vi "Dashboard-Cory.vi"(0 "SensorInputData":T8, 1 "ActuatorInputs":T7, 2 "HMI to Control":T5={"RightDriveValue"=0.0, "LeftDriveValue"=0.0, "Arm Manual "=0.0, "Stacker Manual "=0.0, "Claw Manual "=0.0, "ClawSlightOpenNumber"=0, "Intake Value "=0.0, "Arm States"=enum."4 Tote", "Claw States"=enum."Claw Manual ", "Intake Man. or Sense"=enum."Sensing", "Stacker in Manual?"=FALSE, "Drop Stack? "=FALSE, "Tusk Up Request"=FALSE, "Tusk Down Request"=FALSE, "Inver. Wheels  In Request"=FALSE, "Inverse. Wheels Out Request "=FALSE, "Get Out of Manual Control"=FALSE, "Exit Score State"=FALSE, "DriveStraight Help?"=FALSE, "Stacker Shut Off No."=0, "Stacker Need Off?"=FALSE, "Collecting?"=FALSE, "Go to Hover"=FALSE, "Stack Clamp Lock "=FALSE, "Stack Clamp Unlock "=FALSE, "Claw Intake Value "=0.0, "Stack Clamp Lock No. "=0, "Steal Can (ruin their day?)"=FALSE, "Retract (have mercy?)"=FALSE, "Can Grab No. "=0, "Wench Value to Control "=0.0}, 3 "Stacker to Dashboard":T1={"# of Totes Out"=0, "Stacker State to Index"=enum."Hold", "Stacker Off?"=FALSE, "Stack Clamp Locked?"=FALSE}) -> ()   [LabVIEW 2014]
uses:
  Typedefs/SensorInputData.ctl
  Typedefs/ActuatorInputs.ctl
  Typedefs/HMI_to_Control.ctl
  Typedefs/Arm States.ctl
  Typedefs/ClawStates.ctl
  Typedefs/IntakeWheelSenseOrManual.ctl
  Typedefs/StackerStates.ctl
  Typedefs/StackerToDashboardData.ctl
  <vilib>/Rock Robotics/Network Tables/SD Write Boolean.vi
  <vilib>/Rock Robotics/Network Tables/SD Write Number.vi
  Gensubs/Bert_or_Ernie.vi
  Auton/scriptlib/auto_data.vi
  <vilib>/Rock Robotics/Network Tables/SD Write String Array.vi
panel:
  out "Stack Clamp Locked?":bool
  out "On Bert?":bool
  out "Intake":dbl
  out "Arm":dbl
  out "Stacker":dbl
  out "LeftDrive":dbl
  out "RightDrive":dbl
  out "Stacker Off?":bool
  out "Stacker State to Index":T2=enum."Hold"
  out "Intake See Tote":bool
  out "Claw Manual?":bool=TRUE
  out "Compressor Enabled":bool
  out "Compressor Run":bool
  out "Claw Sees Can":bool
  out "Arm States":T3
  out "Claw States":T4
  in  "MaxSlightOpenNumber":i8
  out "Stacker Manual":bool
  out "# of Totes":u8
  out "Intake Sensing?":bool
  out "ClawOpen%":dbl(slide) scale=0.0..1.0
  out "Tusk":bool
  out "Stacker See Tote":bool
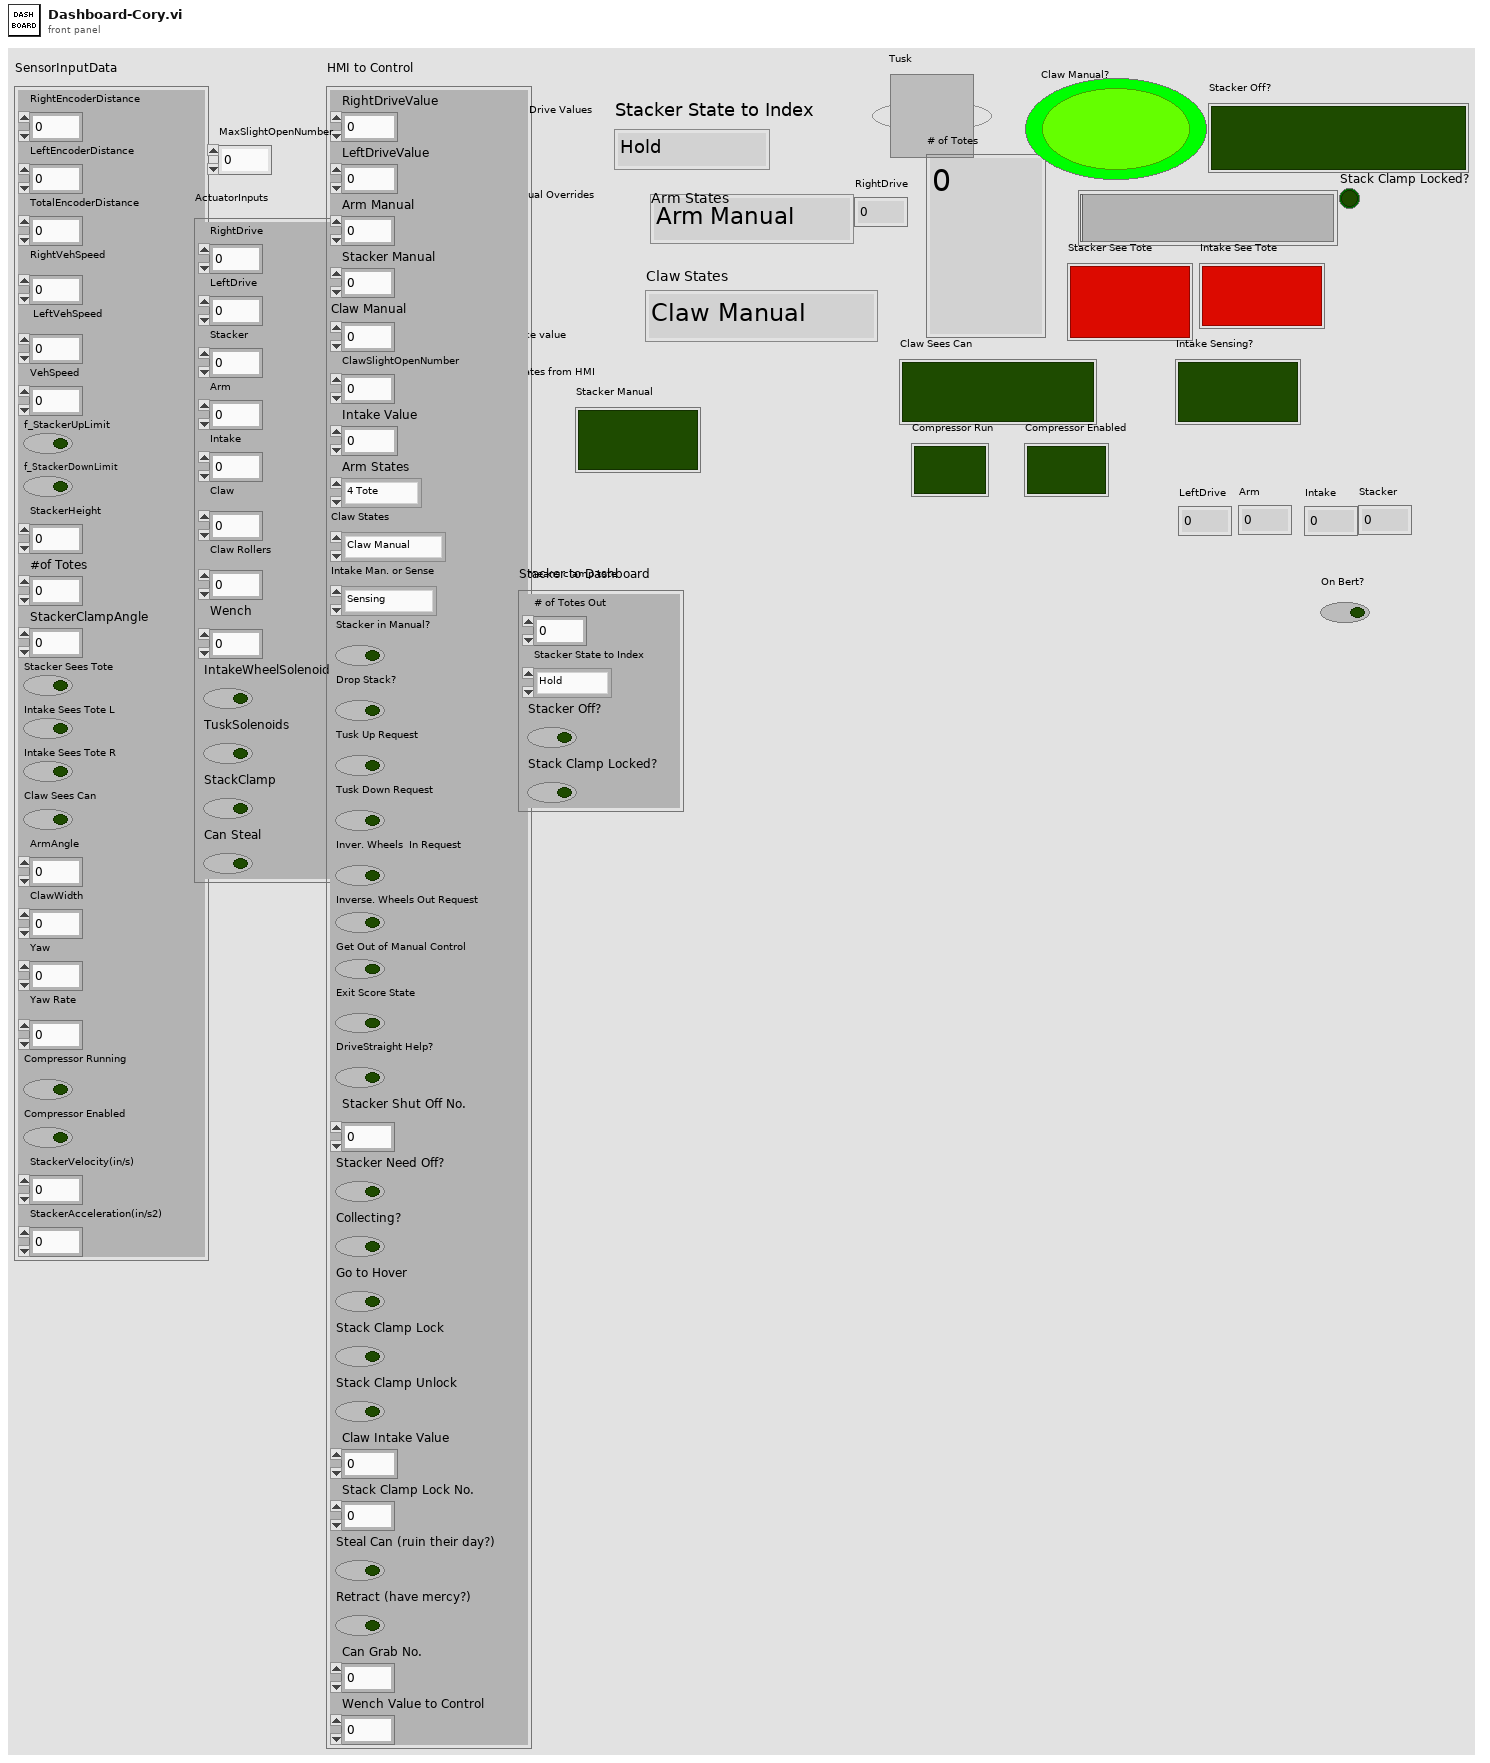
[diagram p1: front panel]
types:
  T1 = typedef "StackerToDashboardData.ctl" = cluster{"# of Totes Out":i32, "Stacker State to Index":T2, "Stacker Off?":bool, "Stack Clamp Locked?":bool}
  T2 = typedef "StackerStates.ctl" = enum16{"Manual ", "Hold", "Hold5", "Hold6", "GetTote", "DropStack", "Hover", "Hover5", "Wait for Up", "DecideHold", "DownTimerPeriod", "Prep Intake for Drop", "Check Arm before 5", "Make Arm ready for 5", "Check Arm before 6", "Make Arm ready for 6", "Delay for 5", "Delay for 6"}
  T3 = typedef "Arm States.ctl" = enum16{"Arm Manual ", "Ground", "Step", "1 Tote", "2 Tote", "3 Tote", "4 Tote", "5 Tote", "6 Tote", "Flip Can Arm", "Grab Can in auto", "Nudge"}
  T4 = typedef "ClawStates.ctl" = enum16{"Claw Manual ", "Claw Open", "Claw Closed", "Claw Slight Open", "Flip Can"}
  T5 = typedef "HMI_to_Control.ctl" = cluster{"RightDriveValue":dbl, "LeftDriveValue":dbl, "Arm Manual ":dbl, "Stacker Manual ":dbl, "Claw Manual ":dbl, "ClawSlightOpenNumber":i8, "Intake Value ":sgl, "Arm States":T3, "Claw States":T4, "Intake Man. or Sense":T6, "Stacker in Manual?":bool, "Drop Stack? ":bool, "Tusk Up Request":bool, "Tusk Down Request":bool, "Inver. Wheels  In Request":bool, "Inverse. Wheels Out Request ":bool, "Get Out of Manual Control":bool, "Exit Score State":bool, "DriveStraight Help?":bool, "Stacker Shut Off No.":i8, "Stacker Need Off?":bool, "Collecting?":bool, "Go to Hover":bool, "Stack Clamp Lock ":bool, "Stack Clamp Unlock ":bool, "Claw Intake Value ":sgl, "Stack Clamp Lock No. ":i8, "Steal Can (ruin their day?)":bool, "Retract (have mercy?)":bool, "Can Grab No. ":i8, "Wench Value to Control ":dbl}
  T6 = typedef "IntakeWheelSenseOrManual.ctl" = enum16{"Sensing", "Manual "}
  T7 = typedef "ActuatorInputs.ctl" = cluster{"RightDrive":dbl, "LeftDrive":dbl, "Stacker":dbl, "Arm":dbl, "Intake":sgl, "Claw":dbl, "Claw Rollers":i8, "Wench":dbl, "IntakeWheelSolenoids":bool, "TuskSolenoids":bool, "StackClamp":bool, "Can Steal":bool}
  T8 = typedef "SensorInputData.ctl" = cluster{"RightEncoderDistance":dbl, "LeftEncoderDistance":dbl, "TotalEncoderDistance":dbl, "RightVehSpeed":dbl, "LeftVehSpeed":dbl, "VehSpeed":dbl, "f_StackerUpLimit":bool, "f_StackerDownLimit":bool, "StackerHeight":dbl, "#of Totes":u8, "StackerClampAngle":dbl, "Stacker Sees Tote":bool, "Intake Sees Tote L":bool, "Intake Sees Tote R":bool, "Claw Sees Can":bool, "ArmAngle":dbl, "ClawWidth":dbl, "Yaw":dbl, "Yaw Rate":dbl, "Compressor Running":bool, "Compressor Enabled":bool, "StackerVelocity(in/s)":dbl, "StackerAcceleration(in/s2)":dbl}
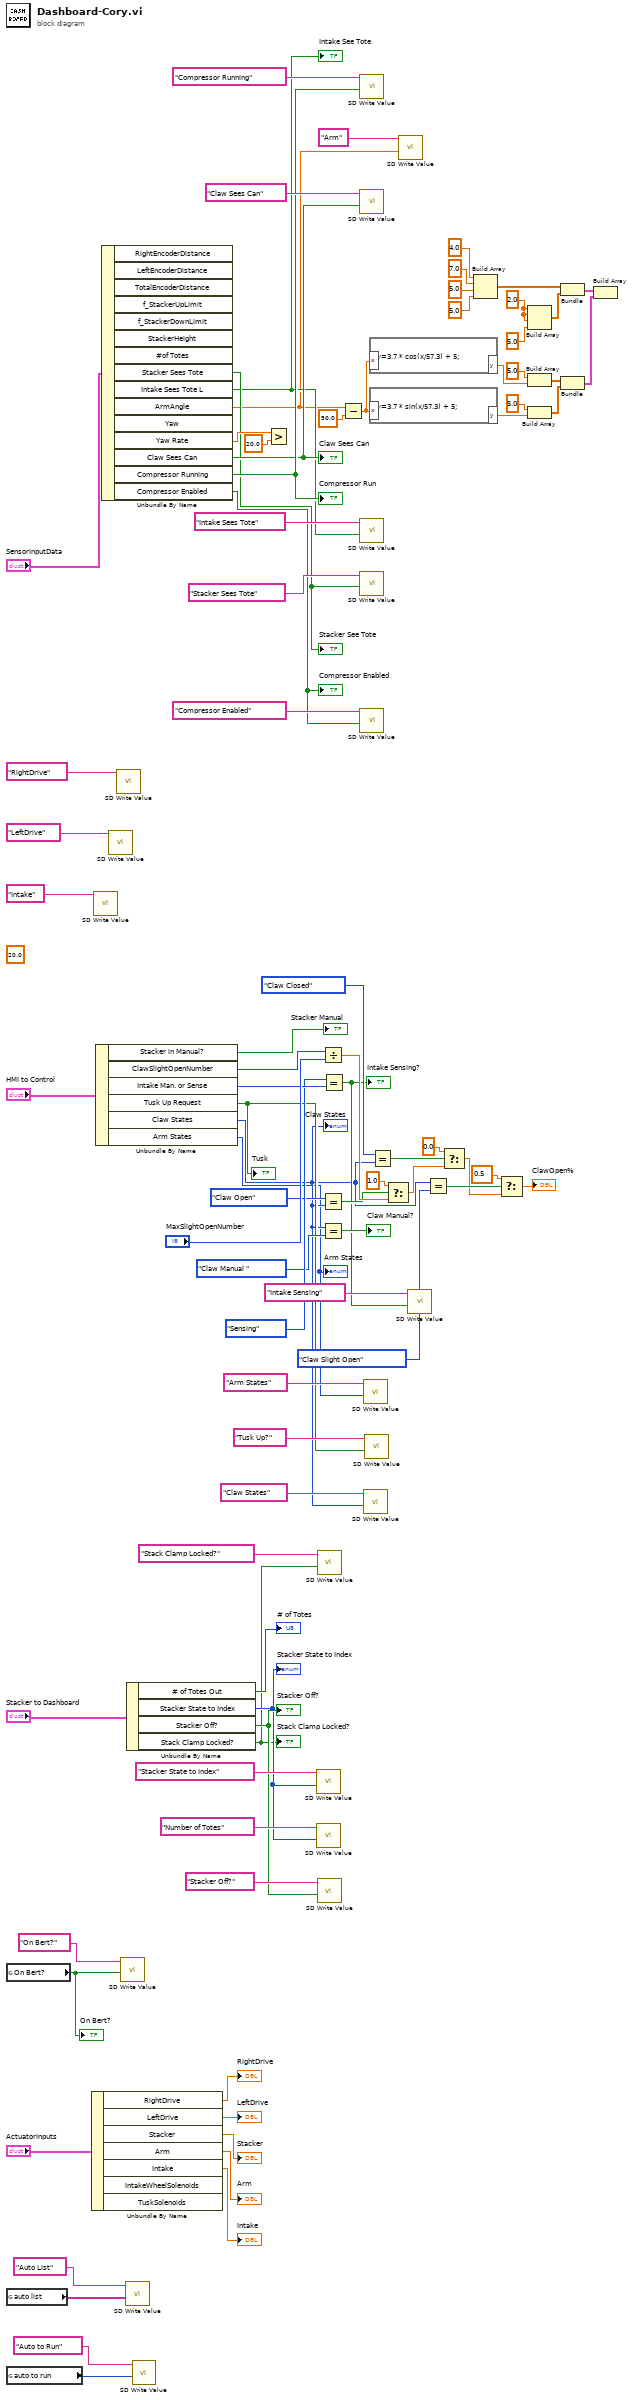
[diagram p0: block diagram]
diagram:
  (unwired) 20.0 ("y")
  w69 = 2.0 ("element")
  n1 = global read "Bert_or_Ernie.vi" "On Bert?"() -> (w17:bool)
  "On Bert?" <- w17
  n2 = global read "auto_data.vi" "auto list"() -> (w3:string[])
  n3 = global read "auto_data.vi" "auto to run"() -> (w4:i8)
  n4 = Unbundle By Name("ActuatorInputs") -> ("RightDrive"=→"RightDrive":dbl, "LeftDrive"=→"LeftDrive":dbl, "Stacker"=→"Stacker":dbl, "Arm"=→"Arm":dbl, "Intake"=→"Intake":sgl)  [unwired: 2 out]
  n5 = call-poly <vilib>:"SD Write Value.vi"("Name"="Intake") -> ()  [unwired: 9 in, 2 out]
  n6 = Unbundle By Name("HMI to Control") -> ("Stacker in Manual?"=→"Stacker Manual":bool, "ClawSlightOpenNumber"=w62:i8, "Intake Man. or Sense"=w60:T6, "Tusk Up Request"=w11:bool, "Claw States"=w10:T4, "Arm States"=w9:T3)
  "Tusk" <- w11
  "Claw States" <- w10
  "Arm States" <- w9
  n7 = Unbundle By Name("SensorInputData") -> ("Stacker Sees Tote"=w7:bool, "Intake Sees Tote L"=w6:bool, "ArmAngle"=w5:dbl, "Yaw Rate"=w63:dbl, "Claw Sees Can"=w13:bool, "Compressor Running"=w15:bool, "Compressor Enabled"=w14:bool)  [unwired: 8 out]
  "Stacker See Tote" <- w7
  "Claw Sees Can" <- w13
  "Compressor Run" <- w15
  "Compressor Enabled" <- w14
  "Intake See Tote" <- w6
  n8 = call-poly <vilib>:"SD Write Value.vi"("Name"="LeftDrive") -> ()  [unwired: 9 in, 2 out]
  n9 = call-poly <vilib>:"SD Write Value.vi"("Name"="RightDrive") -> ()  [unwired: 9 in, 2 out]
  n10 = call-poly <vilib>:"SD Write Value.vi"("Boolean"=w17, "Name"="On Bert?") -> ()  [unwired: 8 in, 2 out]
  n11 = call-poly <vilib>:"SD Write Value.vi"("String Array"=w3, "Name"="Auto List") -> ()  [unwired: 8 in, 2 out]
  n12 = Unbundle By Name("Stacker to Dashboard") -> ("# of Totes Out"=→"# of Totes":i32, "Stacker State to Index"=w8:T2, "Stacker Off?"=w12:bool, "Stack Clamp Locked?"=w2:bool)
  "Stacker State to Index" <- w8
  "Stacker Off?" <- w12
  "Stack Clamp Locked?" <- w2
  n13 = call-poly <vilib>:"SD Write Value.vi"("Numeric"=w4, "Name"="Auto to Run") -> ()  [unwired: 8 in, 2 out]
  n14 = Greater?(x=w63, y=20.0) -> ()  [unwired: 1 out]
  n15 = call-poly <vilib>:"SD Write Value.vi"("Numeric"=w8, "Name"="Stacker State to Index") -> ()  [unwired: 8 in, 2 out]
  n16 = call-poly <vilib>:"SD Write Value.vi"("Numeric"=w8, "Name"="Number of Totes") -> ()  [unwired: 8 in, 2 out]
  n17 = call-poly <vilib>:"SD Write Value.vi"("Boolean"=w2, "Name"="Stack Clamp Locked?") -> ()  [unwired: 8 in, 2 out]
  n18 = call-poly <vilib>:"SD Write Value.vi"("Boolean"=w12, "Name"="Stacker Off?") -> ()  [unwired: 8 in, 2 out]
  n19 = Divide(x=w62, y="MaxSlightOpenNumber") -> (x/y=w56:dbl)
  n20 = Equal?(x=ClawStates."Claw Open", y=w10) -> (x = y?=w54:bool)
  n21 = Equal?(x=w10, y=ClawStates."Claw Manual ") -> (x = y?=→"Claw Manual?":bool)
  n22 = Equal?(x=IntakeWheelSenseOrManual."Sensing", y=w60) -> (x = y?=w16:bool)
  "Intake Sensing?" <- w16
  n23 = Subtract(x=w5, y=50.0) -> (x-y=w80:dbl)
  n24 = call-poly <vilib>:"SD Write Value.vi"("Boolean"=w15, "Name"="Compressor Running") -> ()  [unwired: 8 in, 2 out]
  n25 = call-poly <vilib>:"SD Write Value.vi"("Boolean"=w13, "Name"="Claw Sees Can") -> ()  [unwired: 8 in, 2 out]
  n26 = call-poly <vilib>:"SD Write Value.vi"("Boolean"=w6, "Name"="Intake Sees Tote") -> ()  [unwired: 8 in, 2 out]
  n27 = call-poly <vilib>:"SD Write Value.vi"("Boolean"=w7, "Name"="Stacker Sees Tote") -> ()  [unwired: 8 in, 2 out]
  n28 = call-poly <vilib>:"SD Write Value.vi"("Boolean"=w14, "Name"="Compressor Enabled") -> ()  [unwired: 8 in, 2 out]
  n29 = call-poly <vilib>:"SD Write Value.vi"("Numeric"=w9, "Name"="Arm States") -> ()  [unwired: 8 in, 2 out]
  n30 = call-poly <vilib>:"SD Write Value.vi"("Numeric"=w10, "Name"="Claw States") -> ()  [unwired: 8 in, 2 out]
  n31 = call-poly <vilib>:"SD Write Value.vi"("Boolean"=w11, "Name"="Tusk Up?") -> ()  [unwired: 8 in, 2 out]
  n32 = formula code="y=3.7 * cos(x/57.3) + 5;"("x"=w80) -> ("y"=w85:dbl)
  n33 = formula code="y=3.7 * sin(x/57.3) + 5;"("x"=w80) -> ("y"=w84:dbl)
  n34 = Equal?(x=ClawStates."Claw Closed", y=w10) -> (x = y?=w53:bool)
  n35 = Select(t=1.0, s=w54, f=w56) -> (s? t:f=w55:dbl)
  n36 = call-poly <vilib>:"SD Write Value.vi"("Numeric"=w5, "Name"="Arm") -> ()  [unwired: 8 in, 2 out]
  n37 = call-poly <vilib>:"SD Write Value.vi"("Boolean"=w16, "Name"="Intake Sensing") -> ()  [unwired: 8 in, 2 out]
  n38 = Equal?(x=w10, y=ClawStates."Claw Slight Open") -> (x = y?=w48:bool)
  n39 = Select(t=0.0, s=w53, f=w55) -> (s? t:f=w47:dbl)
  n40 = Build Array(4.0 ("element"), 7.0 ("element"), 5.0 ("element"), 5.0 ("element")) -> (w76:dbl[])
  n41 = Select(t=0.5, s=w48, f=w47) -> (s? t:f=→"ClawOpen%":dbl)
  n42 = Build Array(w69, w69, w69, 5.0 ("element")) -> (w75:dbl[])
  n43 = Build Array(5.0 ("element"), w85) -> (w83:dbl[])
  n44 = Build Array(5.0 ("element"), w84) -> (w82:dbl[])
  n45 = Bundle(w76, w75) -> (w77:cluster{dbl[], dbl[]})  [unwired: 1 in]
  n46 = Bundle(w83, w82) -> (w78:cluster{dbl[], dbl[]})  [unwired: 1 in]
  n47 = Build Array(w77, w78) -> ()  [unwired: 1 out]
